vi "WFDC Read Reference Images.vi"(7 "Scan Positions File Path":path, 11 "Error":errorcluster) -> (8 "Ref Images":T1[](array[typedef]), 15 "Error":errorcluster)   [LabVIEW 2016]
uses:
  <vilib>/vision/Image Controls.llb/IMAQ Image.ctl
  WFDC Controls/WFDC Reference Image Info.ctl
panel:
  out "Initial Z":dbl
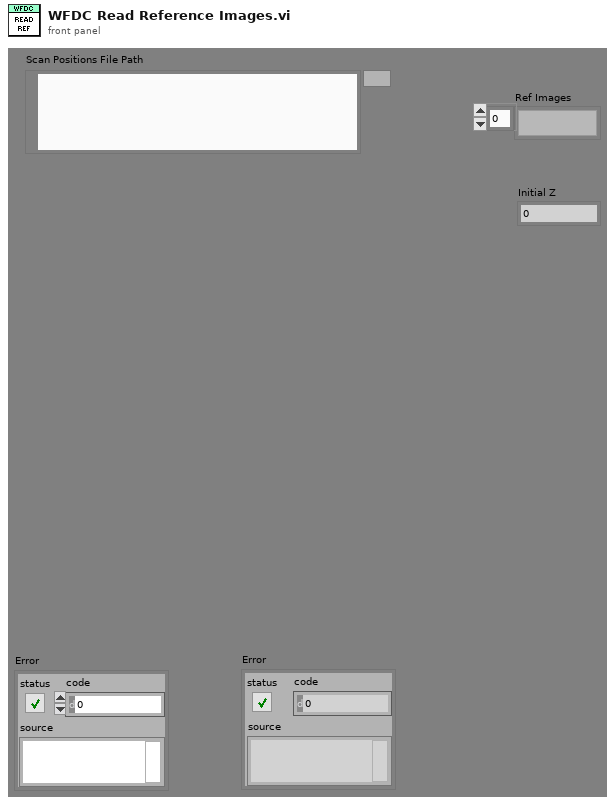
[diagram p1: front panel]
types:
  T1 = typedef "IMAQ Image.ctl" = refnum<image>
  T2 = typedef "WFDC Reference Image Info.ctl" = cluster{"Image Path":path, "Z Position":dbl, "Number of Frames":u32}
  T3 = typedef "Image Type" = u32
  T4 = typedef "TIF Read Image Information.ctl" = cluster{"Byte Order":enum16{"big-endian, network order", "native, host order", "little-endian"}, "Width (pixels)":i32, "Height (pixels)":i32, "Bits per Pixel":u8, "Total Frames":u32, "First Frame Offset (bytes)":u32, "Frame Size (bytes)":u32}
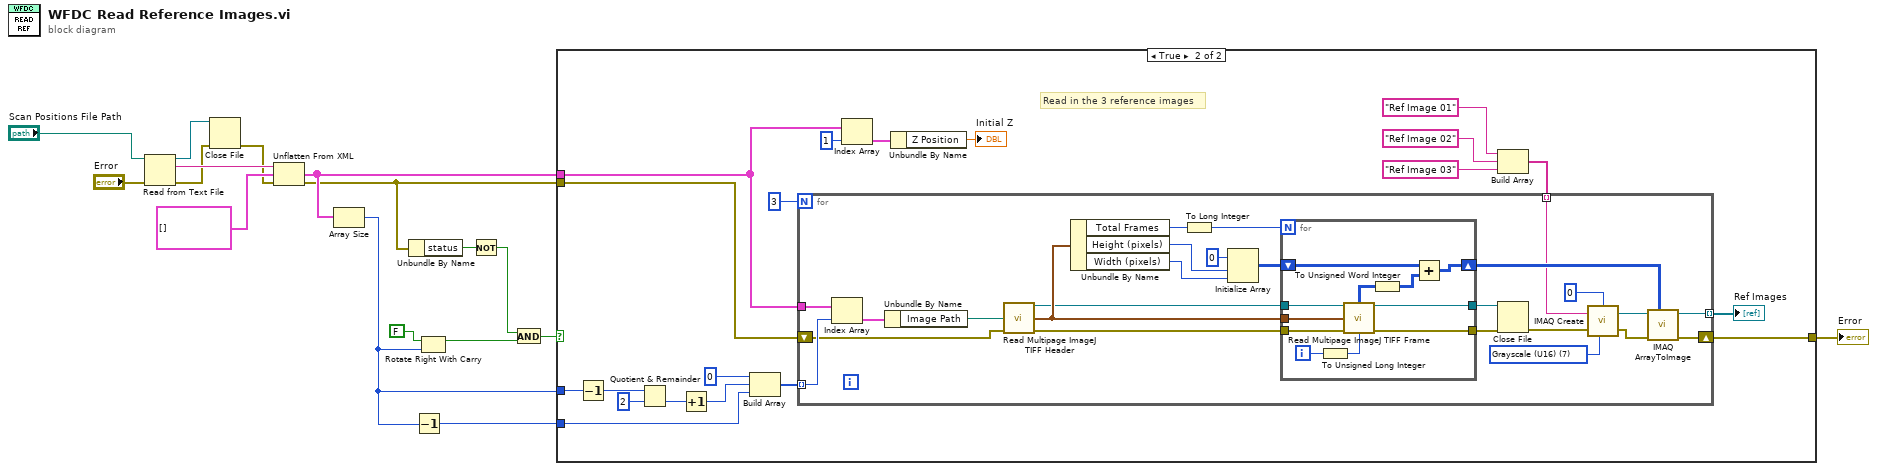
[diagram p0: block diagram]
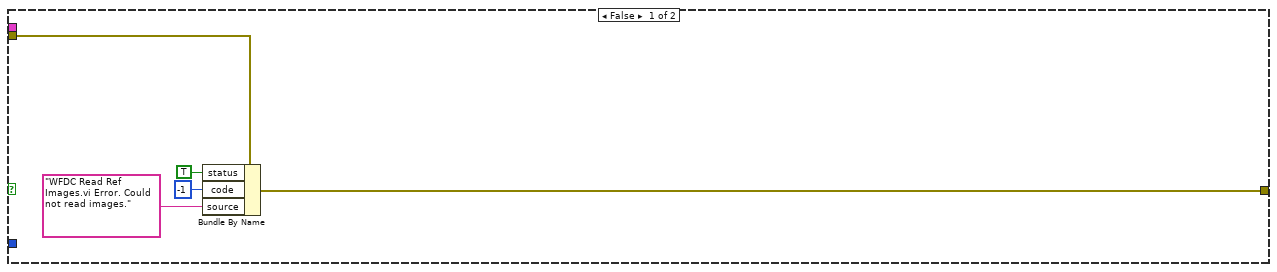
[diagram p2: hidden frame]
diagram:
  n1 = Read from Text File(file (use dialog)="Scan Positions File Path", error in="Error") -> (refnum out=w16:refnum<file>, text=w17:string, error out=w11:errorcluster)  [unwired: 2 in, 1 out]
  n2 = Close File(refnum=w16, error in=w11) -> (error out=w10:errorcluster)  [unwired: 1 out]
  n3 = Unflatten From XML(xml string=w17, type=T2[] [], error in (no error)=w10) -> (value=w13:T2[], error out=w9:errorcluster)
  n4 = Array Size(array=w13) -> (size(s)=w3:i32)
  n5 = Unbundle By Name(w9) -> ("status"=w8:bool)
  n6 = Decrement(x=w3) -> (x-1=w12:i32)
  n7 = Rotate Right With Carry(2:w3, 3:FALSE ("carry")) -> (1:w6:bool)  [unwired: 1 out]
  n8 = Not(x=w8) -> (.not. x?=w7:bool)
  n9 = And(x=w7, y=w6) -> (x .and. y?=w5:bool)
  n10 = case shown="True" w5 {
    tunnel: w3 -> [_ w42]
    tunnel: w13 -> [_ w26]
    tunnel: w12 -> [_ w36]
    tunnel: w9 -> [w22 w28]
    tunnel: [w18 w27] -> w2
    frame False {
      n11 = Bundle By Name(cluster=w22, "status"=TRUE, "code"=-1, "source"="WFDC Read Ref Images.vi Error. Could not read images.") -> (w18:errorcluster)
    }
    frame True {
      # "Read in the 3 reference images"
      n12 = Decrement(x=w42) -> (x-1=w41:i32)
      n13 = Quotient & Remainder(x=w41, y=2) -> (floor(x/y)=w39:i32)  [unwired: 1 out]
      n14 = Increment(x=w39) -> (x+1=w38:i32)
      n15 = Build Array(0 ("element"), w38, w36) -> (w35:i32[])
      n16 = Index Array(array=w26, index=1) -> (element=w24:T2)
      n17 = Unbundle By Name(w24) -> ("Z Position"=→"Initial Z":dbl)
      n18 = Build Array("Ref Image 01" ("Image Name"), "Ref Image 02" ("Image Name"), "Ref Image 03" ("Image Name")) -> (w31:string[])
      n19 = for {
        N: 3 -> [_]
        tunnel: w35 -> [w66] mode=indexing
        tunnel: w26 -> [w67]
        tunnel: [w46] -> w30 mode=indexing
        tunnel: w31 -> [w45] mode=indexing
        shift-right: [w43] -> w27
        shift-left: w28 -> [w44]
        w50 = T3 7 items=["Grayscale (U8)", "Grayscale (I16)", "Grayscale (SGL)", "Complex (CSG)", "RGB (U32)", "HSL (U32)", "RGB (U64)", "Grayscale (U16)"] ("Image Type")
        n20 = Index Array(array=w67, index=w66) -> (element=w65:T2)
        n21 = Unbundle By Name(w65) -> ("Image Path"=w54:path)
        n22 = call "Read Multipage ImageJ TIFF Header.vi"("TIFF Path"=w54, "Error"=w44) -> ("TIF Ref"=w56:refnum<file>, "Image Info"=w58:T4, "Error"=w57:errorcluster)  [unwired: 11 in]
        n23 = Unbundle By Name(w58) -> ("Total Frames"=w59:u32, "Height (pixels)"=w63:i32, "Width (pixels)"=w62:i32)
        n24 = To Long Integer(number=w59) -> (32bit integer=w60:i32)
        n25 = Initialize Array(u16 0 ("element"), w63, w62) -> (w61:u16[][])
        n26 = for {
          N: w60 -> [_]
          tunnel: w56 -> [w78]
          tunnel: w58 -> [w77]
          tunnel: w57 -> [w76]
          shift-right: [w72] -> w47
          shift-left: w61 -> [w73]
          tunnel: [w71] -> w64
          tunnel: [w70] -> w53
          i -> [w75]
          n27 = To Unsigned Long Integer(number=w75) -> (unsigned 32bit integer=w74:u32)
          n28 = call "Read Multipage ImageJ TIFF Frame.vi"("TIF Ref"=w78, "Image Info"=w77, "Error"=w76, "Frame"=w74) -> ("U8 Image"=w69:u8[][], "TIF Ref (Dup)"=w71:refnum<file>, "Error"=w70:errorcluster)  [unwired: 8 in, 1 out]
          n29 = To Unsigned Word Integer(number=w69) -> (unsigned 16bit integer=w68:u16[][])
          n30 = Add(x=w73, y=w68) -> (x+y=w72:u16[][])
        }
        n31 = Close File(refnum=w64, error in=w53) -> (error out=w48:errorcluster)  [unwired: 1 out]
        n32 = call "IMAQ Create"("Border Size"=0, "Image Name"=w45, "Image Type"=w50, "error in (no error)"=w48) -> ("New Image"=w49:T1, "error out"=w52:errorcluster)  [unwired: 1 in]
        n33 = call "IMAQ ArrayToImage"("Image Pixels (U16)"=w47, "error in (no error)"=w52, "Image"=w49) -> ("error out"=w43:errorcluster, "Image Out"=w46:T1)  [unwired: 7 in]
      }
      "Ref Images" <- w30
    }
  }
  "Error" <- w2
